vi "845x_SPI Write.vi"(0 "Device":T1, 1 "Chip Select":u32, 2 "Clock Rate (kHz)":u16=1000, 3 "EEPROM Data Address":u16 format="%.0x", 4 "Data to Write":u8[](array[numeric]), 5 "error in (no error)":errorcluster, 6 "I/O Voltage Level":i32(ring)=33 items=["3.3V"=33, "2.5V"=25, "1.8V"=18, "1.5V"=15, "1.2V"=12], 7 "Data Address Width":enum16{"1 Byte", "2 Byte"}(ring)=enum."2 Byte", 9 "Data Address Endianness":bool=TRUE, 11 "Target Page Size (bytes)":u32=32, 13 "Write Delay Between Pages (ms)":u32=5) -> (19 "error out":errorcluster)   [LabVIEW 2021, in "Communication.lvlib"]
doc: "<B>NOTE: This example is taken from ni845x driver examples located at C:\\Program Files (x86)\\National Instruments\\LabVIEW <version>\\examples\\ni845x\\845xEx.llb. More such examples can be found in the same location.</B>\n\nThis example shows a more generalized way to use the SPI basic API to write data. It allows the user to change the following parameters: page size, write delay, the endianness of the address bytes, and the number of bytes in an address.\n\nThe parameters will have the following effects:\n\nTarget Page Size (bytes): This places an additional constraint on the amount of bytes written. The smaller value will be used, and that number of bytes written.\nWrite Delay Between Pages (ms): This will force a mandatory delay after writing bytes to a device.\nData Address Width: This will allow the user to specify the EEPROM Data Address as either 1 or 2 bytes.\nData Address Endianness: This control will change the ordering of the bytes in the EEPROM Data Address, note that this only has an effect if there are 2 bytes in the address.\n\nFor connection information see the NI-845x Hardware and Software manual and the manual for your specific SPI device."
uses:
  Communication.lvlib
  <vilib>/ni845x/ni845x.llb/ni845xControl.ctl
  <vilib>/ni845x/ni845x.llb/NI-845x SPI Close Configuration Reference.vi
  <resource>/objmgr/NI845x.rc
panel:
  # "See VI Info <Ctrl+I> for more information on how to use this example"
  # "SPI Data"
  # "SPI Slave Configuration"
  # "Device Configuration"
  # "Big Endian"
  # "Little Endian"
  # "NOTE: This example is taken from ni845x driver examples located at C:\\Program Files (x86)\\National Instruments\\LabVIEW <version>\\examples\\ni845x\\845xEx.llb.  More such examples can be found in the same location."
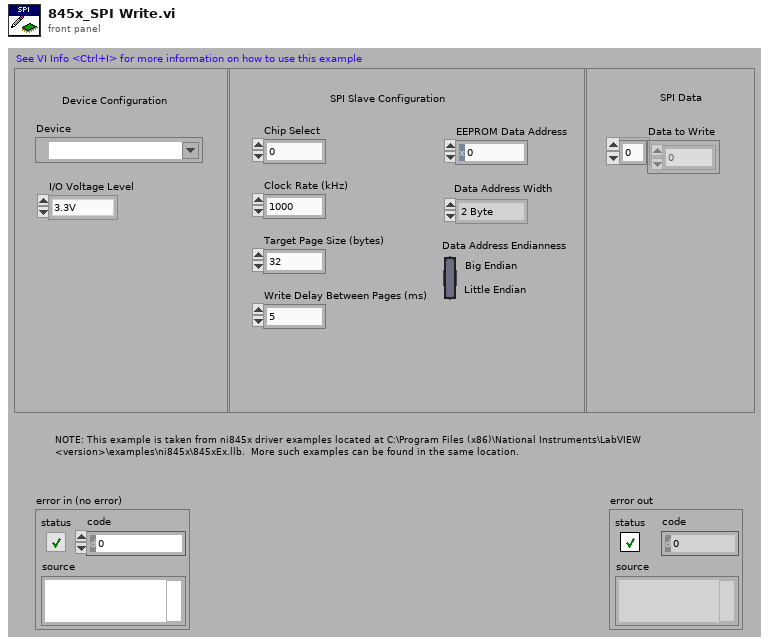
[diagram p1: front panel]
types:
  T1 = typedef "ni845xControl.ctl" = refnum<k21>
  T2 = typedef "ni845xSpiConfiguration.ctl" = refnum<k20>
  T3 = cluster{"EEPROM Address":u16, "Length":u32, "Data Index":u32}[]
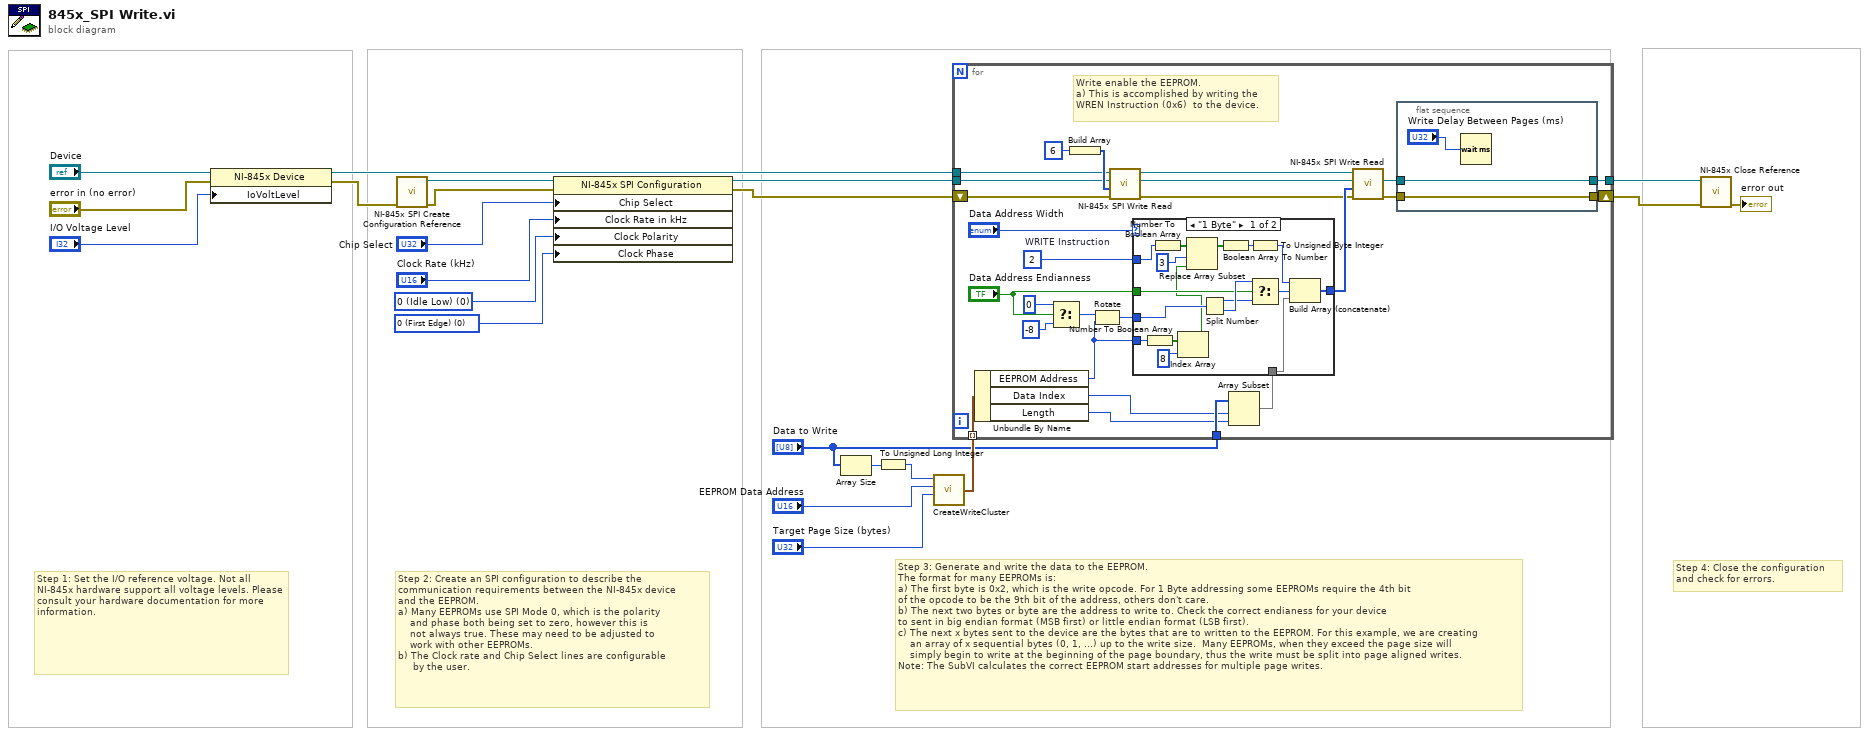
[diagram p0: block diagram]
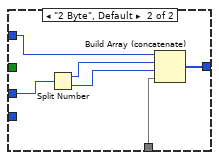
[diagram p2: hidden frame]
diagram:
  w21 = 0 items=["0 (First Edge)", "1 (Second Edge)"] ("Clock Phase")
  w22 = 0 items=["0 (Idle Low)", "1 (Idle High)"] ("Clock Polarity")
  # "Step 1: Set the I/O reference voltage. Not all NI-845x hardware support all voltage levels. Please consult your hardware documentation for more information."
  # "Step 4: Close the configuration \nand check for errors."
  # "Step 2: Create an SPI configuration to describe the \ncommunication requirements between the NI-845x device \nand the EEPROM.\na) Many EEPROMs use SPI Mode 0, which is the polarity \n    and phase both being set to zero, however this is\n    not always true. These may need to be adjusted to\n    work with other EEPROMs.\nb) The Clock rate and Chip Select lines are configurable \n     by the user."
  # "Step 3: Generate and write the data to the EEPROM. \nThe format for many EEPROMs is:\na) The first byte is 0x2, which is the write opcode. For 1 Byte addressing some EEPROMs require the 4th bit \nof the opcode to be the 9th bit of the address, others don't care.\nb) The next two bytes or byte are the address to write to. Check the correct endianess for your device \nto sent in big endian format (MSB first) or little endian format (LSB first).\nc) The next x bytes sent to the device are the bytes that are to written to the EEPROM. For this example, we are creating\n    an array of x sequential bytes (0, 1, ...) up to the write size.  Many EEPROMs, when they exceed the page size will\n    simply begin to write at the beginning of the page boundary, thus the write must be split into page aligned writes.\nNote: The SubVI calculates the correct EEPROM start addresses for multiple page writes."
  n1 = property on="Property Node" class="NI-845x Device"(reference="Device", error in="error in (no error)", "IoVoltLevel"="I/O Voltage Level") -> (reference out=w9:T1, error out=w7:errorcluster)
  n2 = call <vilib>:"NI-845x SPI Create Configuration Reference.vi"("error in (no error)"=w7) -> ("error out"=w17:errorcluster, "spi configuration"=w18:T2)  [unwired: 9 out]
  n3 = property on="Property Node" class="NI-845x SPI Configuration"(reference=w18, error in=w17, "Chip Select"="Chip Select", "Clock Rate in kHz"="Clock Rate (kHz)", "Clock Polarity"=w22, "Clock Phase"=w21) -> (reference out=w10:T2, error out=w11:errorcluster)
  n4 = Array Size(array="Data to Write") -> (size(s)=w2:i32)
  n5 = To Unsigned Long Integer(number=w2) -> (unsigned 32bit integer=w1:u32)
  n6 = call "CreateWriteCluster.vi"("Page Size in Bytes"="Target Page Size (bytes)", "EEPROM Starting Address"="EEPROM Data Address", "Number of Bytes to Write"=w1) -> ("Array of Write Cluster Information"=w13:T3)  [unwired: 1 in]
  n7 = for {
    tunnel: w13 -> [w32] mode=indexing
    tunnel: "Data to Write" -> [w35]
    shift-right: [w41] -> w16
    shift-left: w11 -> [w28]
    tunnel: [w40] -> w15
    tunnel: w10 -> [w26]
    tunnel: w9 -> [w24]
    w48 = u8 2  # WRITE Instruction
    # "Write enable the EEPROM.\na) This is accomplished by writing the \nWREN Instruction (0x6)  to the device."
    n8 = Unbundle By Name(w32) -> ("EEPROM Address"=w31:u16, "Data Index"=w34:u32, "Length"=w33:u32)
    n9 = Select(t=i16 0, s="Data Address Endianness", f=i16 -8) -> (s? t:f=w45:i16)
    n10 = Build Array(u8 6) -> (w30:u8[])
    n11 = Rotate(1:w31, 2:w45) -> (0:w46:u16)
    n12 = call <vilib>:"NI-845x SPI Write Read.vi"("error in (no error)"=w28, "write data"=w30, "spi configuration in"=w26, "device reference in"=w24) -> ("error out"=w27:errorcluster, "spi configuration out"=w25:T2, "device reference out"=w23:T1)  [unwired: 5 out]
    n13 = Array Subset(array=w35, index=w34, length=w33) -> (w36:u8[])
    n14 = case shown="\"1 Byte\"" "Data Address Width" {
      tunnel: [w64 w72] -> w37
      tunnel: w48 -> [w63 w73]
      tunnel: "Data Address Endianness" -> [w65 _]
      tunnel: w46 -> [w62 w71]
      tunnel: w36 -> [w56 w69]
      tunnel: w31 -> [w52 _]
      frame "1 Byte" {
        n15 = Number To Boolean Array(number=w52) -> (Boolean array=w54:bool[])
        n16 = Number To Boolean Array(number=w63) -> (Boolean array=w60:bool[])
        n17 = Index Array(array=w54, index=8) -> (element=w53:bool)
        n18 = Replace Array Subset(array=w60, new element=w53, index=3) -> (w59:bool[])
        n19 = Split Number(x=w62) -> (hi(x)=w66:u8, lo(x)=w67:u8)
        n20 = Boolean Array To Number(Boolean array=w59) -> (number=w58:u32)
        n21 = To Unsigned Byte Integer(number=w58) -> (unsigned 8bit integer=w57:u8)
        n22 = Select(t=w67, s=w65, f=w66) -> (s? t:f=w68:u8)
        n23 = Build Array (concatenate)(w57, w68, w56) -> (w64:u8[])
      }
      frame "2 Byte", Default {
        n24 = Split Number(x=w71) -> (hi(x)=w70:u8, lo(x)=w74:u8)
        n25 = Build Array (concatenate)(w73, w70, w74, w69) -> (w72:u8[])
      }
    }
    n26 = call <vilib>:"NI-845x SPI Write Read.vi"("error in (no error)"=w27, "write data"=w37, "spi configuration in"=w25, "device reference in"=w23) -> ("error out"=w42:errorcluster, "spi configuration out"=w39:T2)  [unwired: 6 out]
    n27 = flat-sequence {
      tunnel: w42 -> [w51]
      tunnel: [w51] -> w41
      tunnel: w39 -> [w50]
      tunnel: [w50] -> w40
      frame #0 {
        n28 = Wait (ms)(milliseconds to wait="Write Delay Between Pages (ms)") -> ()  [unwired: 1 out]
      }
    }
  }
  n29 = call-poly <vilib>:"NI-845x Close Reference.vi"("error in (no error)"=w16, "spi configuration"=w15) -> ("error out"=→"error out":errorcluster)  [unwired: 9 out]
